vi "Get Frequency Shift.vi"(2 "gen":refnum<class "niUSRP Tx DSP v2 FPGA.lvclass">) -> (4 "frequency shift":T1)   [LabVIEW 2025, in "niUSRP Tx DSP v2 FPGA.lvclass"]
uses:
  niUSRP Tx DSP v2 FPGA.lvclass
  <instrlib>/_niInstr/DSP Control/Interface/v1/FPGA/Frequency Shift/IQ 18-bit/Frequency Shift Interface (IQ 18-bit).lvclass
  niUSRP Tx DSP v2 FPGA.lvclass/niUSRP Tx DSP v2 FPGA.ctl
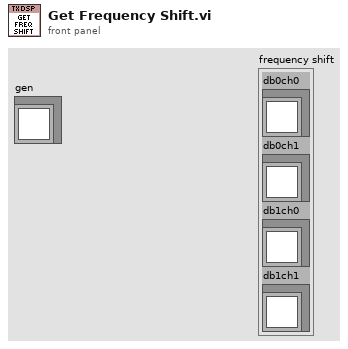
[diagram p1: front panel]
types:
  T1 = cluster{"db0ch0":refnum<class "Frequency Shift Interface (IQ 18-bit).lvclass">, "db0ch1":refnum<class "Frequency Shift Interface (IQ 18-bit).lvclass">, "db1ch0":refnum<class "Frequency Shift Interface (IQ 18-bit).lvclass">, "db1ch1":refnum<class "Frequency Shift Interface (IQ 18-bit).lvclass">}
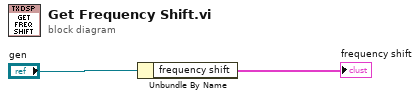
[diagram p0: block diagram]
diagram:
  n1 = Unbundle By Name("gen") -> ("frequency shift"=→"frequency shift":T1)
